vi "User_Panel Hidden.vi"(8 "error in (no error)":errorcluster caption="错误输入（无错误）") -> (0 "error out":errorcluster caption="错误输出")   [LabVIEW 2020]
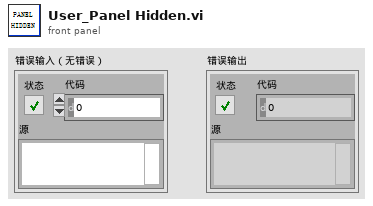
[diagram p1: front panel]
types:
  T1 = enum32{"Invalid", "Standard", "Closed", "Hidden", "Minimized", "Maximized"}
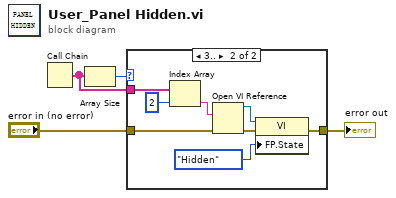
[diagram p0: block diagram]
diagram:
  n1 = Call Chain() -> (call chain=w4:string[])
  n2 = Array Size(array=w4) -> (size(s)=w1:i32)
  n3 = case shown="3.." w1 {
    tunnel: w4 -> [_ w9]
    tunnel: [w5 w7] -> w3
    tunnel: "error in (no error)" -> [w5 w6]
    frame 0, Default {
    }
    frame 3.. {
      n4 = Index Array(array=w9, index=2 ("索引")) -> (element=w13:string)
      n5 = Open VI Reference(vi path=w13, error in (no error)=w6) -> (vi reference=w12:refnum<vi>, error out=w8:errorcluster)  [unwired: 4 in]
      n6 = property class="VI"(reference=w12, error in=w8, "FP.State"=T1."Hidden" ("前面板窗口:状态")) -> (error out=w7:errorcluster)  [unwired: 1 out]
    }
  }
  "error out" <- w3
